vi "Find Test Cases in lvlib.vi"(8 "error in (no error)":errorcluster, 11 "Project Path":path) -> (0 "error out":errorcluster, 2 "Test Class paths":path[](array[path]))   [LabVIEW 2020, in "Test Suite Factory.lvclass"]
uses:
  Test Suite Factory.lvclass
  Core/LUnit Test Case/LUnit Test Case.lvclass
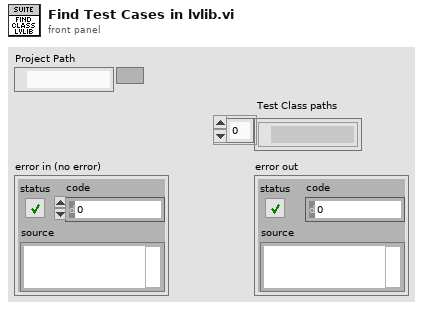
[diagram p1: front panel]
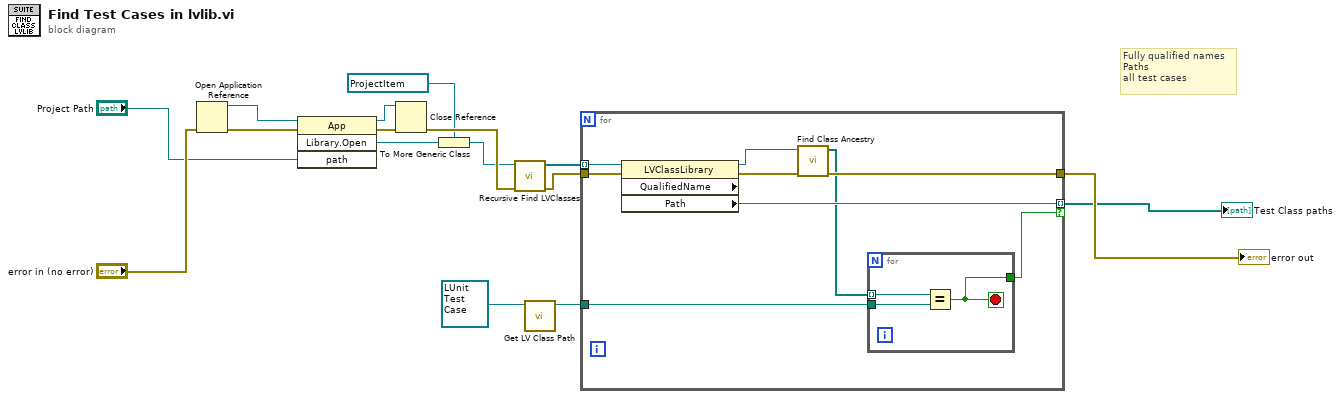
[diagram p0: block diagram]
diagram:
  # "Fully qualified names\nPaths\nall test cases"
  n1 = Open Application Reference(8:"error in (no error)") -> (0:w11:errorcluster, 3:w10:refnum<vi>)  [unwired: 3 in]
  n2 = invoke class="App" method="Library.Open"(reference=w10, error in=w11, "path"="Project Path") -> (reference out=w13:refnum<vi>, error out=w12:errorcluster, "Open Library"=w4:refnum<vi>)  [unwired: 1 in, 1 out]
  n3 = Close Reference(reference=w13, error in (no error)=w12) -> (error out=w6:errorcluster)
  n4 = To More Generic Class(target class=refnum<vi> refnum ("reference"), reference=w4) -> (generic class reference=w3:refnum<vi>)
  n5 = call "Recursive Find LVClasses.vi"("error in (no error)"=w6, "reference"=w3) -> ("error out"=w7:errorcluster, "Class References"=w14:refnum<vi>[])  [unwired: 8 in]
  n6 = call <vilib>:"Get LV Class Path.vi"("object"=refnum<class "LUnit Test Case.lvclass"> refnum ("LUnit Test Case V2.lvclass")) -> ("class path"=w1:path)  [unwired: 9 in, 1 out]
  n7 = for {
    tunnel: w14 -> [w25] mode=indexing
    tunnel: w7 -> [w24]
    tunnel: [w20] -> w16
    tunnel: [w18] -> w8 mode=indexing if=w23
    tunnel: w1 -> [w19]
    n8 = property class="LVClassLibrary" props=["QualifiedName", "Path"](reference=w25, error in=w24) -> (reference out=w22:refnum<vi>, error out=w21:errorcluster, "Path"=w18:path)  [unwired: 1 out]
    n9 = call "Find Class Ancestry.vi"("error in (no error)"=w21, "reference in"=w22) -> ("error out"=w20:errorcluster, "Class Ancestry"=w17:path[])  [unwired: 8 in]
    n10 = for {
      tunnel: w17 -> [w28] mode=indexing
      tunnel: [w27] -> w23
      tunnel: w19 -> [w26]
      stop <- w27 stop-if-true
      n11 = Equal?(x=w28, y=w26) -> (x = y?=w27:bool)
    }
  }
  "error out" <- w16
  "Test Class paths" <- w8
